vi "SymComptModel.vi"() -> ()   [LabVIEW 2014]
uses:
  TypeDefs/SSTestInfoCluster.ctl
  TypeDefs/SignalInfo.ctl
  TypeDefs/Test InfoSS.ctl
  TypeDefs/SampleData.ctl
panel:
  out "DataSamples":dbl[][](array[numeric])
  out "Generated waveforms":waveform(dbl)[](array[waveform])
  in  "DOF":dbl=100.0
  in  "PE %":dbl[](array[numeric])=[0.01282, 0.01308, 0.0123]
  in  "ME %":dbl[](array[numeric])=[0.051, 0.0576, 0.0502]
  in  "E":dbl[][](array[numeric])=[[70.0, 0.0], [70.0, 240.0], [70.0, 120.0]]
  in  "Add Noise":bool
  in  "SSTestInfoCluster":T1={"Signal Information"=[{"Af"=1.0, "Phf"=0.0, "dc"=0.0, "Ah"=9.899, "phh"=0.0}, {"Af"=1.0, "Phf"=-120.0, "dc"=0.0, "Ah"=9.899, "phh"=-120.0}, {"Af"=1.0, "Phf"=120.0, "dc"=0.0, "Ah"=9.899, "phh"=120.0}, {"Af"=0.5, "Phf"=0.0, "dc"=0.0, "Ah"=0.0, "phh"=0.0}, {"Af"=0.5, "Phf"=-120.0, "dc"=0.0, "Ah"=0.0, "phh"=-120.0}, {"Af"=0.5, "Phf"=120.0, "dc"=0.0, "Ah"=0.0, "phh"=120.0}], "Test InfoSS"={"Fc"=60.0, "Interharmonic"=120.0, "Gen rate"=48000.0, "GenSampls"=48000, "SmplIntvl s"=10.0, "sampl rate"=48000.0, "sample mode"=10178, "NI Cycles"=3.0, "Delay"=0.0, "Fit Harmonics"=1, "F0"=60.0, "Fs"=60.0}} {"Test InfoSS"."sample mode" items=["Finite Samples"=10178, "Continuous Samples"=10123, "Hardware Timed Single Point"=12522]}
  out "error out":errorcluster
  in  "error in (no error)":errorcluster
  # "Controls"
  # "Phase"
  # "Mag"
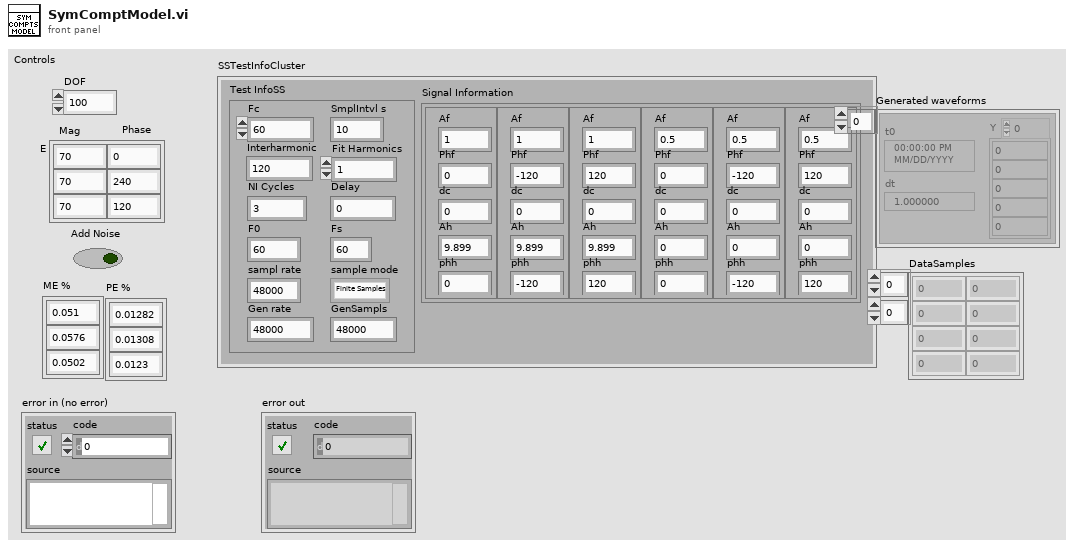
[diagram p1: front panel]
types:
  T1 = typedef "SSTestInfoCluster.ctl" = cluster{"Signal Information":T2, "Test InfoSS":T3}
  T2 = typedef "SignalInfo.ctl" = cluster{"Af":dbl, "Phf":dbl, "dc":dbl, "Ah":dbl, "phh":dbl}[]
  T3 = typedef "Test InfoSS.ctl" = cluster{"Fc":dbl, "Interharmonic":dbl, "Gen rate":dbl, "GenSampls":i32, "SmplIntvl s":dbl, "sampl rate":dbl, "sample mode":i32, "NI Cycles":dbl, "Delay":dbl, "Fit Harmonics":i32, "F0":dbl, "Fs":dbl}
  T4 = typedef "SampleData.ctl" = cluster{"TAI":ext, "Data":dbl[][]}
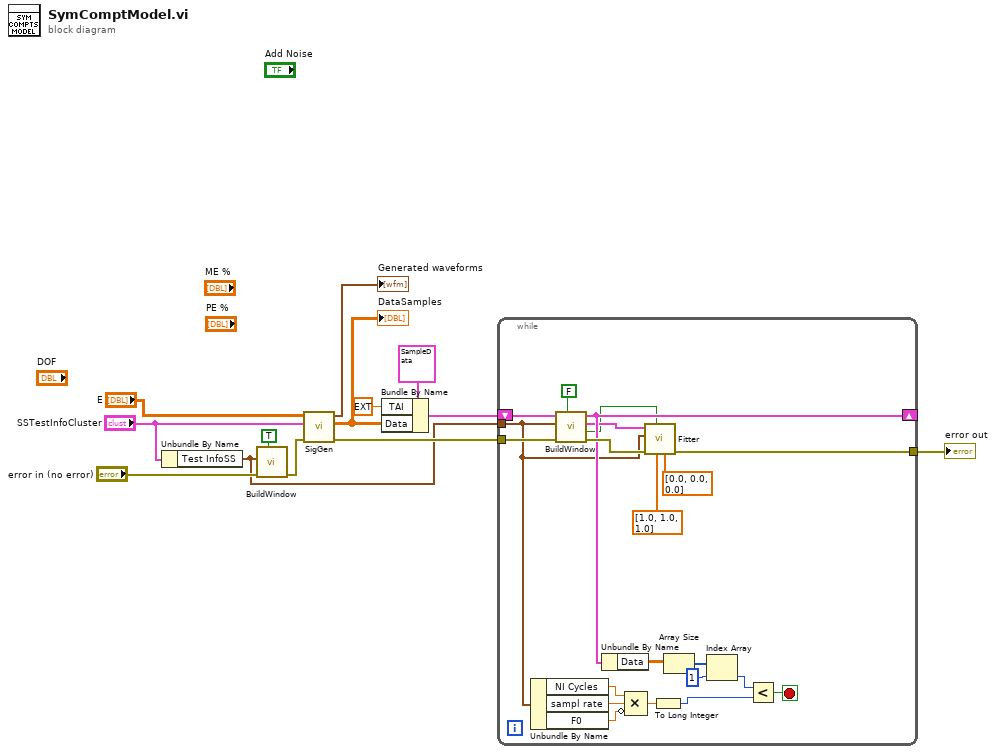
[diagram p0: block diagram]
diagram:
  n1 = Unbundle By Name("SSTestInfoCluster") -> ("Test InfoSS"=w1:T3)
  n2 = call "BuildWindow.vi"("Init (F)"=TRUE, "error in (no error)"="error in (no error)", "Test InfoSS"=w1) -> ("error out"=w5:errorcluster)  [unwired: 5 in, 3 out]
  n3 = call "SigGen.vi"("error in (no error)"=w5, "SSTestInfoCluster"="SSTestInfoCluster", "E"="E") -> ("error out"=w3:errorcluster, "DataSamples"=w10:dbl[][], "Generated waveforms"=→"Generated waveforms":waveform(dbl)[])  [unwired: 6 in]
  "DataSamples" <- w10
  n4 = Bundle By Name(cluster=T4 {"TAI"=3517481187.0499999959, "Data"=array6x2400[14400 elements]} ("SampleData"), "TAI"=ext 0.0, "Data"=w10) -> (w8:T4)
  n5 = while {
    tunnel: w1 -> [w15]
    shift-right: [w19] -> _
    shift-left: w8 -> [w34]
    tunnel: w3 -> [w32]
    tunnel: [w20] -> w2
    stop <- w22 stop-if-true
    n6 = Unbundle By Name(w15) -> ("NI Cycles"=w31:dbl, "sampl rate"=w30:dbl, "F0"=w29:dbl)
    n7 = call "BuildWindow.vi"("Init (F)"=FALSE, "error in (no error)"=w32, "Test InfoSS"=w15, "SampleData"=w34) -> ("error out"=w21:errorcluster, "WindowValid"=w16:bool, "WindowData"=w17:T4, "SampleData"=w19:T4)  [unwired: 4 in]
    n8 = Unbundle By Name(w19) -> ("Data"=w28:dbl[][])
    n9 = Compound Arithmetic op=MULTIPLY(w31, w30, invert w29) -> (w24:dbl)
    n10 = call "Fitter.vi"("Dly Corr"=dbl[] [0.0, 0.0, 0.0], "Mag Corr"=dbl[] [1.0, 1.0, 1.0], "Window Valid"=w16, "error in (no error)"=w21, "Test InfoSS"=w15, "WindowData"=w17) -> ("error out"=w20:errorcluster)  [unwired: 4 in, 1 out]
    n11 = To Long Integer(number=w24) -> (32bit integer=w23:i32)
    n12 = Array Size(array=w28) -> (size(s)=w27:i32[])
    n13 = Index Array(array=w27, index=1) -> (element=w25:i32)
    n14 = Less?(x=w25, y=w23) -> (x < y?=w22:bool)
  }
  "error out" <- w2
